vi "MTMount_getNextSample_BalancingDrives.vi"(8 "error in (no error)":errorcluster, 11 "Balancing_Drives_Ctl":T1) -> (0 "error out":errorcluster, 2 "function return":i32, 3 "Balancing_Drives_Ctl out":T1)   [LabVIEW 2018, in "SALLV_MTMount.lvlib"]
doc: "int MTMount_shm_getNextSample_Balancing_DrivesLV(MTMount_Balancing_DrivesLV *Balancing_Drives_Ctl );"
uses:
  SALLV_MTMount.lvlib
  DataTypes/Balancing_Drives.ctl
  SALLV_MTMount.so
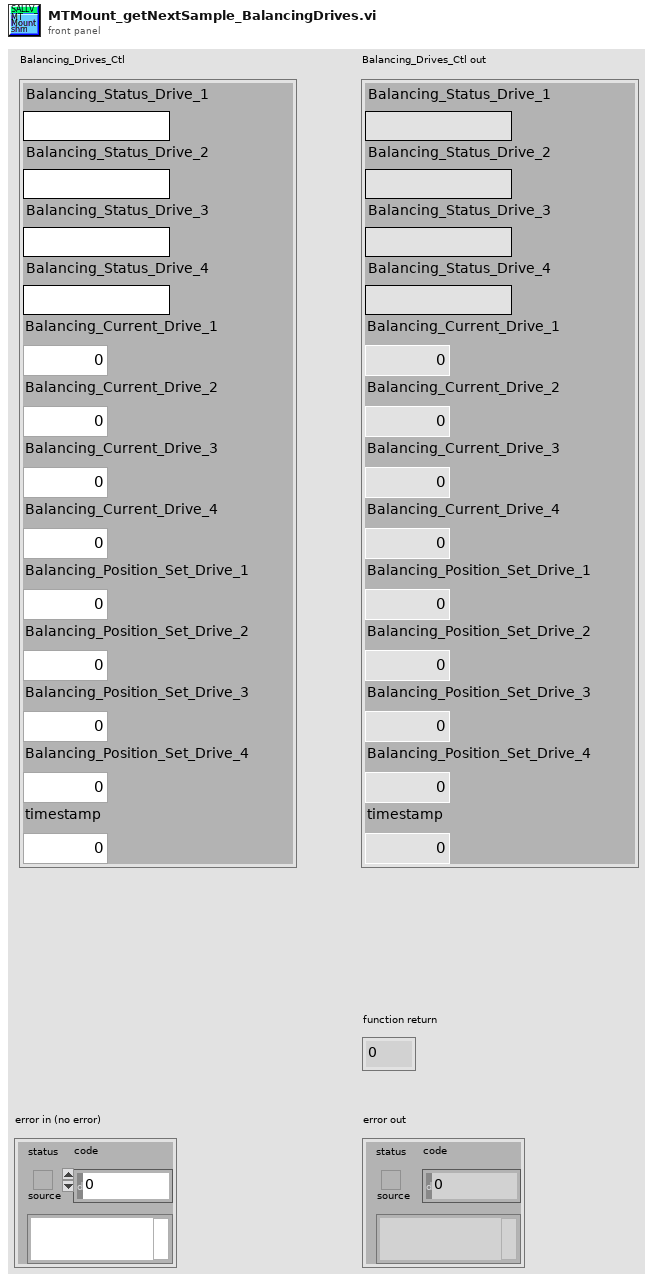
[diagram p1: front panel]
types:
  T1 = typedef "SALLV_MTMount.lvlib/Balancing_Drives.ctl" = cluster{"Balancing_Status_Drive_1":string, "Balancing_Status_Drive_2":string, "Balancing_Status_Drive_3":string, "Balancing_Status_Drive_4":string, "Balancing_Current_Drive_1":dbl, "Balancing_Current_Drive_2":dbl, "Balancing_Current_Drive_3":dbl, "Balancing_Current_Drive_4":dbl, "Balancing_Position_Set_Drive_1":dbl, "Balancing_Position_Set_Drive_2":dbl, "Balancing_Position_Set_Drive_3":dbl, "Balancing_Position_Set_Drive_4":dbl, "timestamp":dbl}
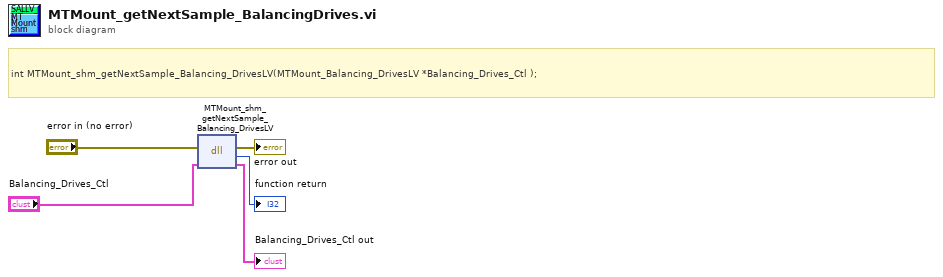
[diagram p0: block diagram]
diagram:
  # "int MTMount_shm_getNextSample_Balancing_DrivesLV(MTMount_Balancing_DrivesLV *Balancing_Drives_Ctl );"
  n1 = dll-call lib="home/ttsai/Document/salApiMTMount/SALLV_MTMount/SALLV_MTMount.*" fn="MTMount_shm_getNextSample_Balancing_DrivesLV"(error in="error in (no error)", "Balancing_Drives_Ctl"="Balancing_Drives_Ctl") -> (error out=→"error out":errorcluster, →"function return":i32, "Balancing_Drives_Ctl"=→"Balancing_Drives_Ctl out":T1)  [unwired: 2 in, 1 out]
